vi "DQtoABC_UnitaryMagnitude_src.vi"(0 "direct":sgl format="%#_30g", 5 "quadrature":sgl format="%#_30g", 7 "theta":sgl) -> (4 "A":sgl format="%#_32g", 6 "B":sgl, 8 "C":sgl, 10 "alpha":sgl format="%#_30g", 13 "sinx":sgl, 14 "cosx":sgl, 15 "beta":sgl format="%#_30g")   [LabVIEW 2015]
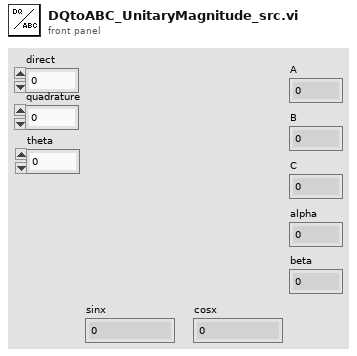
[diagram p1: front panel]
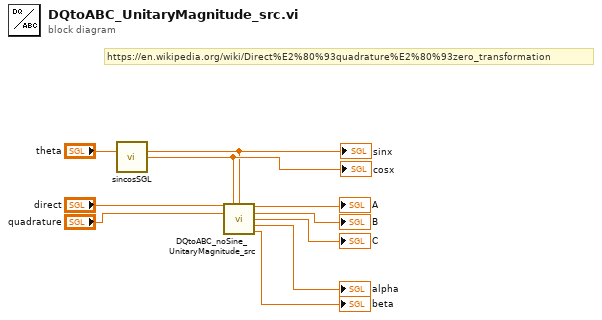
[diagram p0: block diagram]
diagram:
  # "https://en.wikipedia.org/wiki/Direct%E2%80%93quadrature%E2%80%93zero_transformation"
  n1 = call "sincosSGL.vi"("x"="theta") -> ("sinx"=w1:sgl, "cosx"=w2:sgl)  [unwired: 13 in]
  "sinx" <- w1
  "cosx" <- w2
  n2 = call "DQtoABC_noSine_UnitaryMagnitude_src.vi"("d"="direct", "cos"=w2, "sin"=w1, "q"="quadrature") -> ("a"=→"A":sgl, "b"=→"B":sgl, "c"=→"C":sgl, "alpha"=→"alpha":sgl, "beta"=→"beta":sgl)  [unwired: 7 in]
